vi "PTScanner.ProcState.vi"(0 "i ref in":refnum<vi>, 2 "state timeout":i32=-1, 4 "state":string, 5 "error in":errorcluster) -> (14 "i ref out":refnum<vi>, 18 "next state":string, 19 "error out":errorcluster)   [LabVIEW 2014, in "PTScanner.lvlib"]
uses:
  PTScanner.lvlib
  CSCore/CSSystem/CoreDefs/CoreDefs.error_type.ctl
  CSCore/BaseSM/BaseSM.lvlib
  CSCore/CSSystem/CoreLib/CoreLib.lvlib
  CSCore/BaseProcess/BaseProcess.lvlib
  CSCore/CSSystem/CSSystemLib/CSSystemLib.lvlib
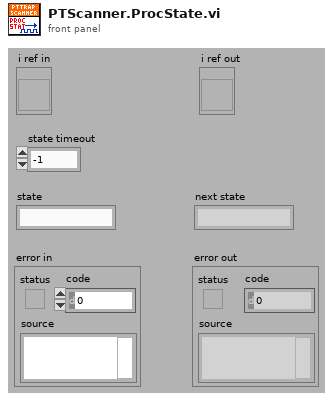
[diagram p1: front panel]
types:
  T1 = typedef "CoreDefs.error_type.ctl" = enum16{"no error", "can't load process", "can't unload process", "process does not exist", "can't install process", "can't remove process", "unknown function", "time out", "can't execute function", "duplicate queue name", "super not found", "caller queue invalid", "can't ping process", "unknown error", "VISA Error", "VISA timeout", "GPIB timeout", "GPIB error", "communication error", "data type mismatch", "can't read data from OPC server", "can't write data to OPC server", "OET error", "function not implemented", "process already exists", "invalid Shared Variable name", "error writing Shared Variable", "error reading Shared Variable", "invalid client name", "corrupt database", "unknown class", "call not authorized", "parameter out of range", "OET timeout: can't get data to modify", "invalid queue name", "requested operation incompatible with current state", "event undefined", "event disabled", "state undefined", "caller is not a friend", "EventBuilder: bad eventID", "EventBuilder: no DAQ devices", "a thread must not stop itself", "UNUSED ELEMENT4", "DiscArchiver: eventData incomplete", "DiscArchiver: eventData does not belong to run", "DiscArchiver: can't open file", "DiscArchiver: can't write to file", "DiscArchiver: available disc space low", "can't acquire semaphore", "error reading data from database", "notifier object is not existing", "can't register process", "can't unregister process", "illegal event type", "object disabled", "object already exists", "can't change state", "Instrument not found", "no connection to remote node", "invalid reference", "N/A", "UNUSED ELEMENT 1", "element not found", "illegal TCP/IP connection detected", "object does not exist", "invalid access ID", "unknown CS system", "invalid privilige", "unsupported data type", "unsupported server type", "IO server already exists", "Shared Variable already exists"}
  T2 = typedef "PTScanner.lvlib/PTScanner.i attribute.ctl" = cluster{"Object cmds":T3[], "Steps":cluster{"Finished":bool, "cmd setup":T4[]}[], "curStep":i32, "DIM IDs":cluster{"AllFinished":i32, "Finished":i32, "curStep":i32, "nofSteps":i32, "NomValues":i32[], "1D-Min":i32, "1D-Max":i32, "Dimensions":i32, "MaxDimensions":i32, "ScanedDeviceNames":i32[]}, "All Finished":bool, "DIMs in use":string[], "Running":bool, "Scan Delay":u32, "loop":bool, "Paused":bool, "Formed":bool}
  T3 = typedef "PTScanner.lvlib/PTScanner.obj parameters.ctl" = cluster{"object":string, "DIM address":string, "method":string, "data descriptor":string, "method parameters":cluster{"Name":string, "Descr":string, "Value":string, "Value?":bool}[], "Call Mode":enum16{"Simple DIM", "Synchronous"}, "actValue":dbl, "Centroid":dbl, "Minus Delta":dbl, "Plus Delta":dbl, "increment":dbl, "DIM Status":cluster{"no link":bool, "quality":i32, "Time Stamp":timestamp}, "range":dbl, "DIMChannelIndex":i32}
  T4 = typedef "PTScanner.lvlib/PTScanner.step obj parameters.ctl" = cluster{"obj index":i32, "nomValue":dbl, "fulfilled":bool}
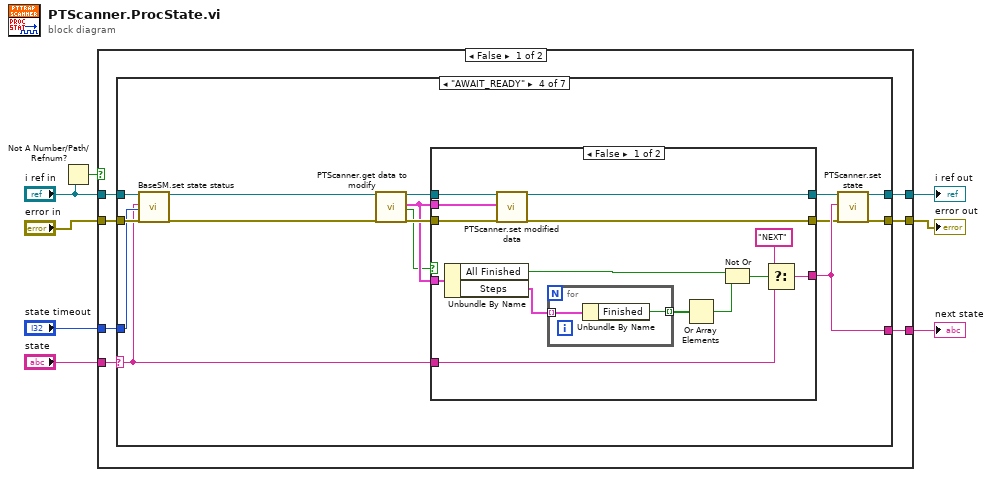
[diagram p0: block diagram]
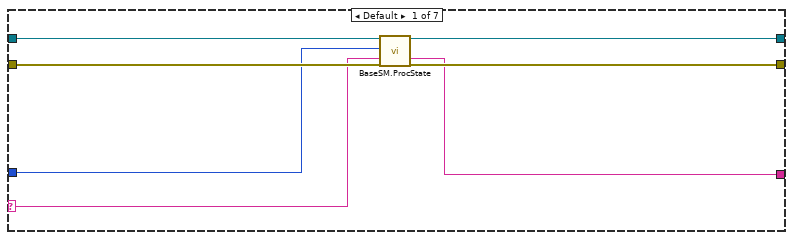
[diagram p2: hidden frame]
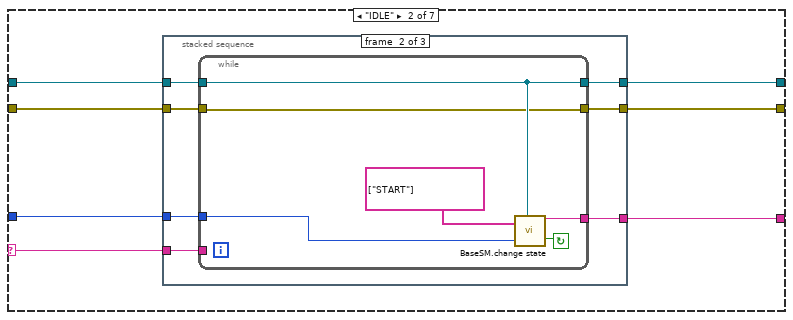
[diagram p3: hidden frame]
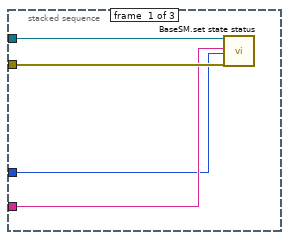
[diagram p4: hidden frame]
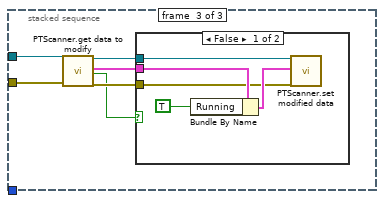
[diagram p5: hidden frame]
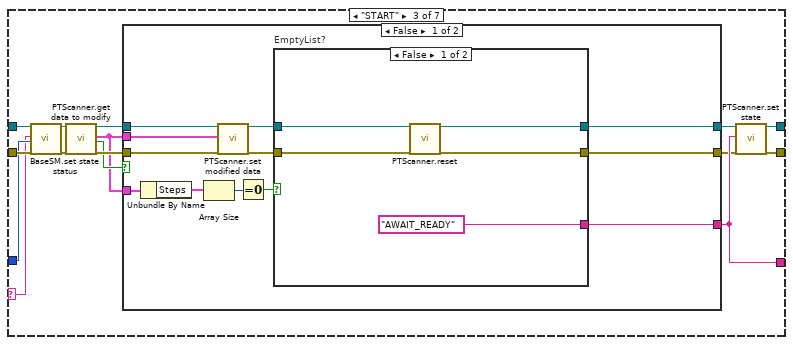
[diagram p7: hidden frame]
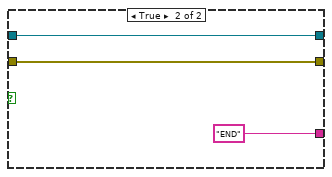
[diagram p8: hidden frame]
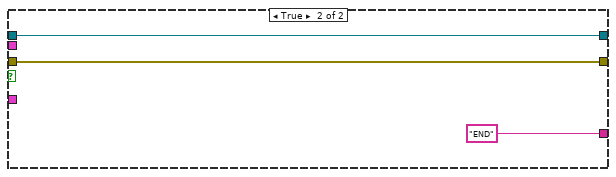
[diagram p9: hidden frame]
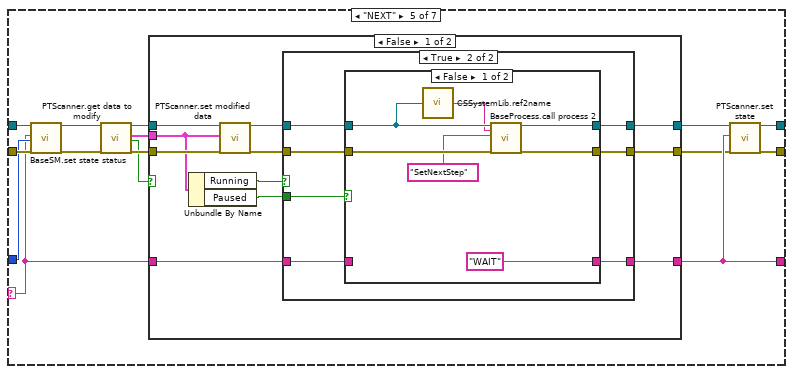
[diagram p11: hidden frame]
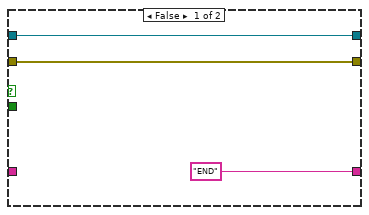
[diagram p12: hidden frame]
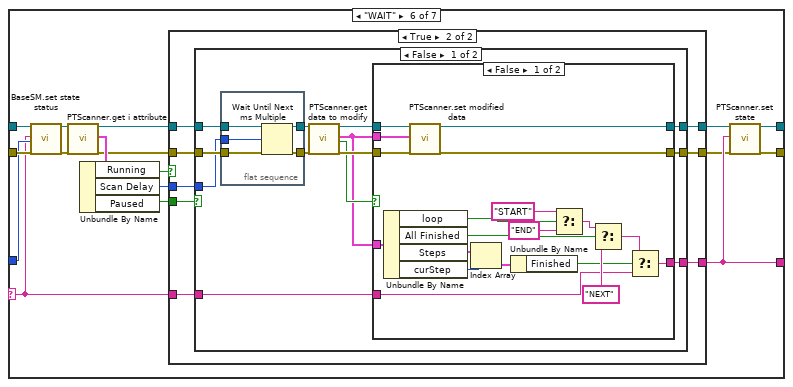
[diagram p15: hidden frame]
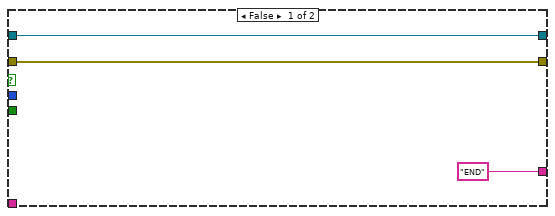
[diagram p16: hidden frame]
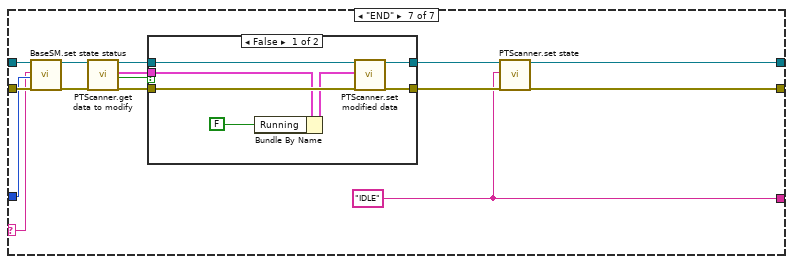
[diagram p19: hidden frame]
diagram:
  n1 = Not A Number/Path/Refnum?(number/path/refnum="i ref in") -> (NaN/Path/Refnum?=w2:bool)
  n2 = case shown="False" w2 {
    tunnel: "i ref in" -> [w15 w275]
    tunnel: [w14 w275] -> w8
    tunnel: "state" -> [w13 w272]
    tunnel: [w12 w272] -> w6
    tunnel: "state timeout" -> [w11 _]
    tunnel: "error in" -> [w10 _]
    tunnel: [w9 w273] -> w3
    frame False {
      n3 = case shown="\"AWAIT_READY\"" w13 {
        selector: w13 -> [w17 w26 w65 w102 w130 w187 w257]
        tunnel: w15 -> [w22 w29 w71 w109 w143 w194 w261]
        tunnel: [w21 w25 w67 w105 w141 w192 w251] -> w14
        tunnel: [w16 w23 w64 w103 w139 w190 w248] -> w12
        tunnel: w11 -> [w18 w27 w70 w108 w142 w193 w260]
        tunnel: w10 -> [w20 w28 w72 w110 w144 w195 w262]
        tunnel: [w19 w24 w66 w104 w140 w191 w249] -> w9
        frame Default {
          n4 = call "BaseSM.ProcState.vi"("i ref in"=w22, "state timeout [ms]"=w18, "state"=w17, "error in (no error)"=w20) -> ("i ref out"=w21:refnum<vi>, "next state"=w16:string, "error out"=w19:errorcluster)  [unwired: 13 in]
        }
        frame "IDLE" {
          n5 = stacked-sequence {
            tunnel: w26 -> [w31 w40 _]
            tunnel: [_ w39 _] -> w23
            tunnel: w29 -> [w33 w37 w52]
            tunnel: [_ w36 _] -> w25
            tunnel: w27 -> [w30 w38 _]
            tunnel: w28 -> [w32 w34 w51]
            tunnel: [_ w35 _] -> w24
            frame #0 {
              n6 = call "BaseSM.set state status.vi"("i ref in"=w33, "stateStatus"=w31, "ms timeout (10000)"=w30, "error in (no error)"=w32) -> ()  [unwired: 13 in, 3 out]
            }
            frame #1 {
              n7 = while {
                tunnel: w38 -> [w44]
                tunnel: [w46] -> w39
                tunnel: w40 -> [_]
                tunnel: w37 -> [w42]
                tunnel: [w42] -> w36
                tunnel: [w41] -> w35
                tunnel: w34 -> [w41]
                stop <- w45 continue-if-true
                n8 = call "BaseSM.change state.vi"("allowed next states"=string[] ["START"], "wait time [ms]"=w44, "i ref in"=w42) -> ("next state"=w46:string, "continue loop"=w45:bool)  [unwired: 13 in, 2 out]
              }
            }
            frame #2 {
              n9 = call "PTScanner.get data to modify.vi"("i ref in"=w52, "error in (no error)"=w51) -> ("i ref out"=w50:refnum<vi>, "i attribute"=w49:T2, "timed out"=w47:bool, "error out"=w48:errorcluster)  [unwired: 14 in]
              n10 = case shown="False" w47 {
                tunnel: w50 -> [w57 _]
                tunnel: w49 -> [w56 _]
                tunnel: w48 -> [w53 _]
                frame False {
                  n11 = Bundle By Name(cluster=w56, "Running"=TRUE) -> (w55:T2)
                  n12 = call "PTScanner.set modified data.vi"("i ref in"=w57, "CLASS.i attribute"=w55, "error in (no error)"=w53) -> ()  [unwired: 15 in, 2 out]
                }
                frame True {
                }
              }
            }
          }
        }
        frame "START" {
          n13 = call "BaseSM.set state status.vi"("i ref in"=w71, "stateStatus"=w65, "ms timeout (10000)"=w70, "error in (no error)"=w72) -> ("i ref out"=w69:refnum<vi>, "error out"=w68:errorcluster)  [unwired: 13 in, 1 out]
          n14 = call "PTScanner.get data to modify.vi"("i ref in"=w69, "error in (no error)"=w68) -> ("i ref out"=w63:refnum<vi>, "i attribute"=w58:T2, "timed out"=w59:bool, "error out"=w62:errorcluster)  [unwired: 14 in]
          n15 = case shown="False" w59 {
            tunnel: [w84 "END"] -> w64
            tunnel: w58 -> [w83 _]
            tunnel: w63 -> [w77 w95]
            tunnel: w62 -> [w76 w94]
            tunnel: [w79 w95] -> w61
            tunnel: [w78 w94] -> w60
            tunnel: w58 -> [w73 _]
            frame False {
              n16 = Unbundle By Name(w83) -> ("Steps"=w80:cluster{"Finished":bool, "cmd setup":T4[]}[])
              n17 = Array Size(array=w80) -> (size(s)=w82:i32)
              n18 = call "PTScanner.set modified data.vi"("i ref in"=w77, "CLASS.i attribute"=w73, "error in (no error)"=w76) -> ("i ref out"=w74:refnum<vi>, "error out"=w75:errorcluster)  [unwired: 15 in]
              n19 = Equal To 0?(x=w82) -> (x = 0?=w81:bool)
              n20 = case "EmptyList?" shown="False" w81 {
                tunnel: ["AWAIT_READY" ("next state") "END" ("next state")] -> w84
                tunnel: w74 -> [w88 w91]
                tunnel: [w86 w91] -> w79
                tunnel: w75 -> [w87 w90]
                tunnel: [w85 w90] -> w78
                frame False {
                  n21 = call "PTScanner.reset.vi"("i ref in"=w88, "error in (no error)"=w87) -> ("i ref out"=w86:refnum<vi>, "error out"=w85:errorcluster)  [unwired: 16 in]
                }
                frame True {
                }
              }
            }
            frame True {
            }
          }
          n22 = call "PTScanner.set state.vi"("i ref in"=w61, "state"=w64, "error in (no error)"=w60) -> ("i ref out"=w67:refnum<vi>, "error out"=w66:errorcluster)  [unwired: 15 in]
        }
        frame "AWAIT_READY" {
          n23 = call "BaseSM.set state status.vi"("i ref in"=w109, "stateStatus"=w102, "ms timeout (10000)"=w108, "error in (no error)"=w110) -> ("i ref out"=w107:refnum<vi>, "error out"=w106:errorcluster)  [unwired: 13 in, 1 out]
          n24 = call "PTScanner.get data to modify.vi"("i ref in"=w107, "error in (no error)"=w106) -> ("i ref out"=w101:refnum<vi>, "i attribute"=w99:T2, "timed out"=w98:bool, "error out"=w100:errorcluster)  [unwired: 14 in]
          n25 = case shown="False" w98 {
            tunnel: w99 -> [w124 _]
            tunnel: [w122 w127] -> w103
            tunnel: w102 -> [w121 w127]
            tunnel: w101 -> [w115 w129]
            tunnel: w100 -> [w114 w128]
            tunnel: w99 -> [w113 _]
            tunnel: [w112 w129] -> w97
            tunnel: [w111 w128] -> w96
            frame False {
              n26 = Unbundle By Name(w124) -> ("All Finished"=w118:bool, "Steps"=w120:cluster{"Finished":bool, "cmd setup":T4[]}[])
              n27 = call "PTScanner.set modified data.vi"("i ref in"=w115, "CLASS.i attribute"=w113, "error in (no error)"=w114) -> ("i ref out"=w112:refnum<vi>, "error out"=w111:errorcluster)  [unwired: 15 in]
              n28 = for {
                tunnel: w120 -> [w126] mode=indexing
                tunnel: [w125] -> w119 mode=indexing
                n29 = Unbundle By Name(w126) -> ("Finished"=w125:bool)
              }
              n30 = Or Array Elements(Boolean array=w119) -> (logical OR=w117:bool)
              n31 = Not Or(1:w117, 2:w118) -> (0:w116:bool)
              n32 = Select(t="NEXT", s=w116, f=w121) -> (s? t:f=w122:string)
            }
            frame True {
            }
          }
          n33 = call "PTScanner.set state.vi"("i ref in"=w97, "state"=w103, "error in (no error)"=w96) -> ("i ref out"=w105:refnum<vi>, "error out"=w104:errorcluster)  [unwired: 15 in]
        }
        frame "NEXT" {
          n34 = call "BaseSM.set state status.vi"("i ref in"=w143, "stateStatus"=w130, "ms timeout (10000)"=w142, "error in (no error)"=w144) -> ("i ref out"=w136:refnum<vi>, "error out"=w135:errorcluster)  [unwired: 13 in, 1 out]
          n35 = call "PTScanner.get data to modify.vi"("i ref in"=w136, "error in (no error)"=w135) -> ("i ref out"=w134:refnum<vi>, "i attribute"=w132:T2, "timed out"=w131:bool, "error out"=w133:errorcluster)  [unwired: 14 in]
          n36 = case shown="False" w131 {
            tunnel: [w155 w176] -> w139
            tunnel: [w154 w178] -> w138
            tunnel: [w153 w177] -> w137
            tunnel: w134 -> [w151 w178]
            tunnel: w133 -> [w149 w177]
            tunnel: w132 -> [w147 _]
            tunnel: w130 -> [w145 w176]
            frame False {
              n37 = Unbundle By Name(w147) -> ("Running"=w152:bool, "Paused"=w146:bool)
              n38 = call "PTScanner.set modified data.vi"("i ref in"=w151, "CLASS.i attribute"=w147, "error in (no error)"=w149) -> ("i ref out"=w150:refnum<vi>, "error out"=w148:errorcluster)  [unwired: 15 in]
              n39 = case shown="True" w152 {
                tunnel: ["END" ("next state") w161] -> w155
                tunnel: [w157 w162] -> w154
                tunnel: [w156 w165] -> w153
                tunnel: w150 -> [w157 w164]
                tunnel: w148 -> [w156 w163]
                tunnel: w146 -> [_ w160]
                tunnel: w145 -> [_ w159]
                frame False {
                }
                frame True {
                  n40 = case shown="False" w160 {
                    tunnel: [w172 w174] -> w165
                    tunnel: w164 -> [w171 w175]
                    tunnel: w163 -> [w170 w174]
                    tunnel: [w169 w175] -> w162
                    tunnel: ["WAIT" ("next state") w173] -> w161
                    tunnel: w159 -> [_ w173]
                    frame False {
                      n41 = call "CSSystemLib.ref2name.vi"("obj refnum"=w171) -> ("name"=w166:string)
                      n42 = call "BaseProcess.call process 2.vi"("i ref in"=w171, "Object"=w166, "Selector"="SetNextStep" ("data string"), "error in (no error)"=w170) -> ("i ref out"=w169:refnum<vi>, "error out"=w172:errorcluster)  [unwired: 14 in]
                    }
                    frame True {
                    }
                  }
                }
              }
            }
            frame True {
            }
          }
          n43 = call "PTScanner.set state.vi"("i ref in"=w138, "state"=w139, "error in (no error)"=w137) -> ("i ref out"=w141:refnum<vi>, "error out"=w140:errorcluster)  [unwired: 15 in]
        }
        frame "WAIT" {
          n44 = call "BaseSM.set state status.vi"("i ref in"=w194, "stateStatus"=w187, "ms timeout (10000)"=w193, "error in (no error)"=w195) -> ("i ref out"=w186:refnum<vi>, "error out"=w185:errorcluster)  [unwired: 13 in, 1 out]
          n45 = call "PTScanner.get i attribute.vi"("i ref in"=w186, "error in (no error)"=w185) -> ("i ref out"=w182:refnum<vi>, "i attribute"=w184:T2, "error out"=w181:errorcluster)  [unwired: 15 in]
          n46 = Unbundle By Name(w184) -> ("Running"=w183:bool, "Scan Delay"=w180:u32, "Paused"=w179:bool)
          n47 = case shown="True" w183 {
            tunnel: ["END" w206] -> w190
            tunnel: [w197 w205] -> w189
            tunnel: [w196 w204] -> w188
            tunnel: w187 -> [_ w203]
            tunnel: w182 -> [w197 w202]
            tunnel: w181 -> [w196 w201]
            tunnel: w180 -> [_ w200]
            tunnel: w179 -> [_ w199]
            frame False {
            }
            frame True {
              n48 = case shown="False" w199 {
                tunnel: [w219 w245] -> w206
                tunnel: [w218 w247] -> w205
                tunnel: [w217 w246] -> w204
                tunnel: w203 -> [w216 w245]
                tunnel: w202 -> [w215 w247]
                tunnel: w201 -> [w214 w246]
                tunnel: w200 -> [w213 _]
                frame False {
                  n49 = flat-sequence {
                    tunnel: w215 -> [w222]
                    tunnel: w214 -> [w221]
                    tunnel: [w222] -> w207
                    tunnel: [w221] -> w208
                    tunnel: w213 -> [w220]
                    frame #0 {
                      n50 = Wait Until Next ms Multiple(millisecond multiple=w220) -> ()  [unwired: 1 out]
                    }
                  }
                  n51 = call "PTScanner.get data to modify.vi"("i ref in"=w207, "error in (no error)"=w208) -> ("i ref out"=w212:refnum<vi>, "i attribute"=w209:T2, "timed out"=w210:bool, "error out"=w211:errorcluster)  [unwired: 14 in]
                  n52 = case shown="False" w210 {
                    tunnel: [w230 w242] -> w219
                    tunnel: w209 -> [w241 _]
                    tunnel: w212 -> [w240 w244]
                    tunnel: [w229 w244] -> w218
                    tunnel: w211 -> [w239 w243]
                    tunnel: [w228 w243] -> w217
                    tunnel: w209 -> [w238 _]
                    tunnel: w216 -> [w227 w242]
                    frame False {
                      n53 = Unbundle By Name(w241) -> ("loop"=w226:bool, "All Finished"=w235:bool, "Steps"=w234:cluster{"Finished":bool, "cmd setup":T4[]}[], "curStep"=w233:i32)
                      n54 = call "PTScanner.set modified data.vi"("i ref in"=w240, "CLASS.i attribute"=w238, "error in (no error)"=w239) -> ("i ref out"=w229:refnum<vi>, "error out"=w228:errorcluster)  [unwired: 15 in]
                      n55 = Index Array(array=w234, index=w233) -> (element=w232:cluster{"Finished":bool, "cmd setup":T4[]})
                      n56 = Unbundle By Name(w232) -> ("Finished"=w231:bool)
                      n57 = Select(t="START", s=w226, f="END") -> (s? t:f=w223:string)
                      n58 = Select(t=w223, s=w235, f="NEXT") -> (s? t:f=w236:string)
                      n59 = Select(t=w236, s=w231, f=w227) -> (s? t:f=w230:string)
                    }
                    frame True {
                    }
                  }
                }
                frame True {
                }
              }
            }
          }
          n60 = call "PTScanner.set state.vi"("i ref in"=w189, "state"=w190, "error in (no error)"=w188) -> ("i ref out"=w192:refnum<vi>, "error out"=w191:errorcluster)  [unwired: 15 in]
        }
        frame "END" {
          w248 = "IDLE"
          n61 = call "BaseSM.set state status.vi"("i ref in"=w261, "stateStatus"=w257, "ms timeout (10000)"=w260, "error in (no error)"=w262) -> ("i ref out"=w259:refnum<vi>, "error out"=w258:errorcluster)  [unwired: 13 in, 1 out]
          n62 = call "PTScanner.get data to modify.vi"("i ref in"=w259, "error in (no error)"=w258) -> ("i ref out"=w254:refnum<vi>, "i attribute"=w256:T2, "timed out"=w255:bool, "error out"=w253:errorcluster)  [unwired: 14 in]
          n63 = case shown="False" w255 {
            tunnel: w253 -> [w269 w270]
            tunnel: w254 -> [w268 w271]
            tunnel: w256 -> [w267 _]
            tunnel: [w264 w271] -> w252
            tunnel: [w263 w270] -> w250
            frame False {
              n64 = Bundle By Name(cluster=w267, "Running"=FALSE ("Pause?")) -> (w265:T2)
              n65 = call "PTScanner.set modified data.vi"("i ref in"=w268, "CLASS.i attribute"=w265, "error in (no error)"=w269) -> ("i ref out"=w264:refnum<vi>, "error out"=w263:errorcluster)  [unwired: 15 in]
            }
            frame True {
            }
          }
          n66 = call "PTScanner.set state.vi"("i ref in"=w252, "state"=w248, "error in (no error)"=w250) -> ("i ref out"=w251:refnum<vi>, "error out"=w249:errorcluster)  [unwired: 15 in]
        }
      }
    }
    frame True {
      n67 = call "CoreLib.my to LV error.vi"("ErrorTypes"=CoreDefs.error_type."invalid reference") -> ("myErrorCluster"=w273:errorcluster)  [unwired: 17 in, 1 out]
    }
  }
  "i ref out" <- w8
  "next state" <- w6
  "error out" <- w3
